vi "Drive Controller.vi"(8 "error in":errorcluster) -> ()   [LabVIEW 2017]
doc: "This VI executes continuously carrying out the current operation and responding to updates or new operation requests. It will often contain the timing or control code that is difficult to place directly in TeleOp. This VI generally opens all sensors and motors and isolates the rest of the robot code from knowing implementation details of how the operations are carried out."
uses:
  <vilib>/Rock Robotics/WPI/Framework/Completion Status.ctl
  Drive Setpoints.ctl
  Drive Operations.ctl
  <vilib>/Rock Robotics/WPI/SafetyOutput/WPI_SafetyOutputConfigMenu.ctl
  <vilib>/Rock Robotics/SystemInterfaces/DIO/FPGA_DIOPWMChannel.ctl
  <vilib>/Rock Robotics/WPI/RobotDrive/WPI_RobotDriveOpen4MotorWithTalonSRX.vi
  Framework/Robot Global Data.vi
  <vilib>/addons/control/pid/pid.llb/PID (DBL).vi
  <vilib>/Rock Robotics/Network Tables/NT Write Numeric Array.vi
  <vilib>/addons/control/pid/NI_PID_pid.lvlib
  <vilib>/Rock Robotics/WPI/ThirdParty/Sensors/ADIS16448 IMU/ADIS16448_IMU.lvlib
panel:
  in  "Interactive Values":T1
  in  "Buttons":cluster{"Execute Cmd":bool, "Abort Cmd":bool}
  out "Command Timing":cluster{"Start Time (ms)":u32, "Iterations":i32}
  out "Status":T3
  out "Setpoints":T4(graph)
  out "Current\nCmd":string
  # "Tip: The graph shows the motor setpoints. It may also be helpful to observe inputs and sensor values.\nYou may also want to display tuning or debugging controls."
  # "Interactive Command: You may fill in the settings for a command\nand schedule it with the Execute button. You can observe and abort\nany command while fine tuning the code for the controller."
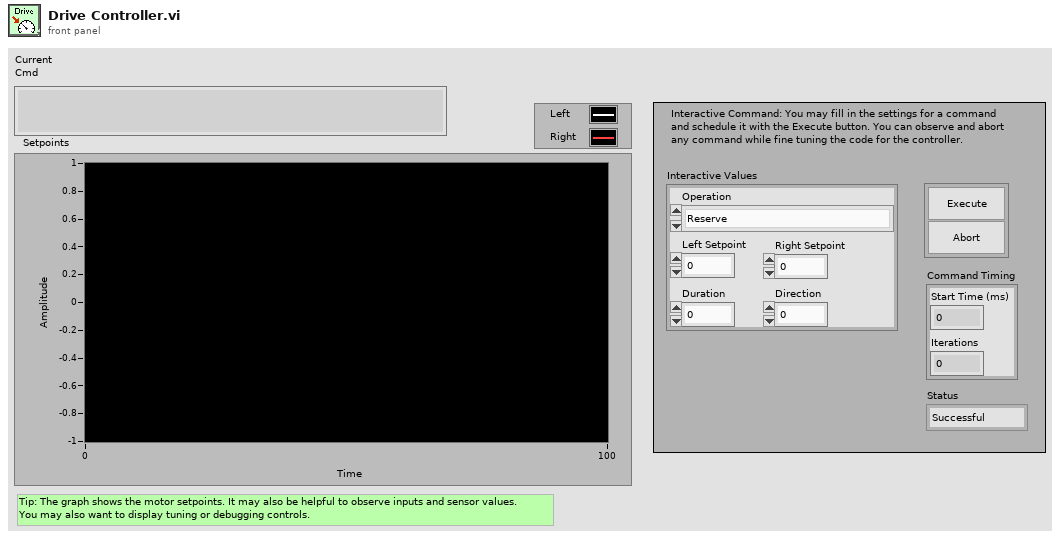
[diagram p1: front panel]
types:
  T1 = typedef "Drive Setpoints.ctl" = cluster{"Operation":T2, "Left Setpoint":dbl, "Right Setpoint":dbl, "Duration":dbl, "Direction":dbl}
  T2 = typedef "Drive Operations.ctl" = enum16{"Reserve", "Read Current", "Immediate", "Drive for Time", "Drive for Distance", "Drive Straight", "Left Turn", "Right Turn", "180 degree Turn", "360 degree Turn"}
  T3 = typedef "Completion Status.ctl" = enum16{"Successful", "Aborted", "Incomplete"}
  T4 = cluster{"Left Setpoint":dbl, "Right Setpoint":dbl}
  T5 = typedef "FPGA_DIOPWMChannel.ctl" = enum8{"PWM 0", "PWM 1", "PWM 2", "PWM 3", "PWM 4", "PWM 5", "PWM 6", "PWM 7", "PWM 8", "PWM 9", "PWM MXP 0", "PWM MXP 1", "PWM MXP 2", "PWM MXP 3", "PWM MXP 4", "PWM MXP 5", "PWM MXP 6", "PWM MXP 7", "PWM MXP 8", "PWM MXP 9", "Invalid"}
  T6 = typedef "WPI_SafetyOutputConfigMenu.ctl" = enum16{"Enable", "Disable"}
  T7 = typedef "WPI_RobotDriveDevRef.ctl" = cluster{"DevStatus":errorcluster, "Motors[]":T8[], "Square Inputs":bool, "Max Output":dbl}
  T8 = typedef "WPI_MotorControlDeviceRef.ctl" = cluster{"DeviceStatus":errorcluster, "Type":T9, "PWM":cluster{"PWM Channel":T5, "DeadBand":T10}, "CAN":cluster{"Device Number":u8, "SetOutput VI Ref":variant, "GetOutput VI Ref":variant, "Enable VI Ref":variant, "Disable VI Ref":variant, "Data":variant}, "Invert":bool, "DIO PWM":cluster{"PWM \"Enable\" Channel":T5, "DIOChannel":T11, "PWM Rate":dbl}}
  T9 = typedef "WPI_MotorControlType.ctl" = enum16{"PWM", "CAN", "DIO PWM"}
  T10 = typedef "WPI_PWMDeadband.ctl" = cluster{"Name":string, "maxPositivePwm":i32, "minPositivePwm":i32, "centerPwm":i32, "maxNegativePwm":i32, "minNegativePwm":i32, "angularRange":u16}
  T11 = typedef "FPGA_DIOChannel.ctl" = enum8{"DIO 0", "DIO 1", "DIO 2", "DIO 3", "DIO 4", "DIO 5", "DIO 6", "DIO 7", "DIO 8", "DIO 9", "DIO MXP 0", "DIO MXP 1", "DIO MXP 2", "DIO MXP 3", "DIO MXP 4", "DIO MXP 5", "DIO MXP 6", "DIO MXP 7", "DIO MXP 8", "DIO MXP 9", "DIO MXP 10", "DIO MXP 11", "DIO MXP 12", "DIO MXP 13", "DIO MXP 14", "DIO MXP 15", "SPI Port CS1", "SPI Port CS2", "SPI Port CS3", "SPI Port MISO", "SPI Port MOSI", "Invalid"}
  T12 = typedef "Command Status Info.ctl" = cluster{"Name":string, "Status":T3, "notifier out":T13}
  T13 = typedef "Completion Notifier.ctl" = refnum<notifier>
  T14 = cluster{"SubSystem Data":T1, cluster{"Start Time (ms)":u32, "Iterations":i32}, cluster{"Command Info":T12, "Description":string, "Default Command":T1, "queue out":refnum<queue>, "Subsystem Name":string}}
  T15 = typedef "ADIS16448_IMU.lvlib/ADI_IMU_ADIS16448_IMUDevRef.ctl" = cluster{"DevStatus":errorcluster, "Handle":i32, "SPI Bus":T16, "Device Found":bool, "Device Ready":bool, "Yaw Axis":enum16{"X", "Y", "Z"}, "AHRS Algorithm":enum16{"Complementary", "Madgwick"}, "Serial":u16, "Lot ID 2":u16, "Lot ID 1":u16, "Bytes Per Sample":u16, "Calibrate On Open?":bool}
  T16 = typedef "spi_bus.ctl" = enum16{"SPI On-Board, CS0", "SPI On-Board, CS1", "SPI On-Board, CS2", "SPI On-Board, CS3", "SPI MXP", "Invalid"}
  T17 = cluster{"proportional gain (Kc)":dbl, "integral time (Ti, min)":dbl, "derivative time (Td, min)":dbl}
  T18 = cluster{"X Angle":dbl, "Y Angle":dbl, "Z Angle":dbl}
  T19 = cluster{"SubSystem Data":T1, cluster{"Start Time (ms)":u32, "Iterations":i32}, "Default Command Arguments":cluster{"Command Info":T12, "Description":string, "Default Command":T1, "queue out":refnum<queue>, "Subsystem Name":string}}
  T20 = cluster{"Don't move motors while reserved":dbl, "Don't move motors while reserved":dbl}
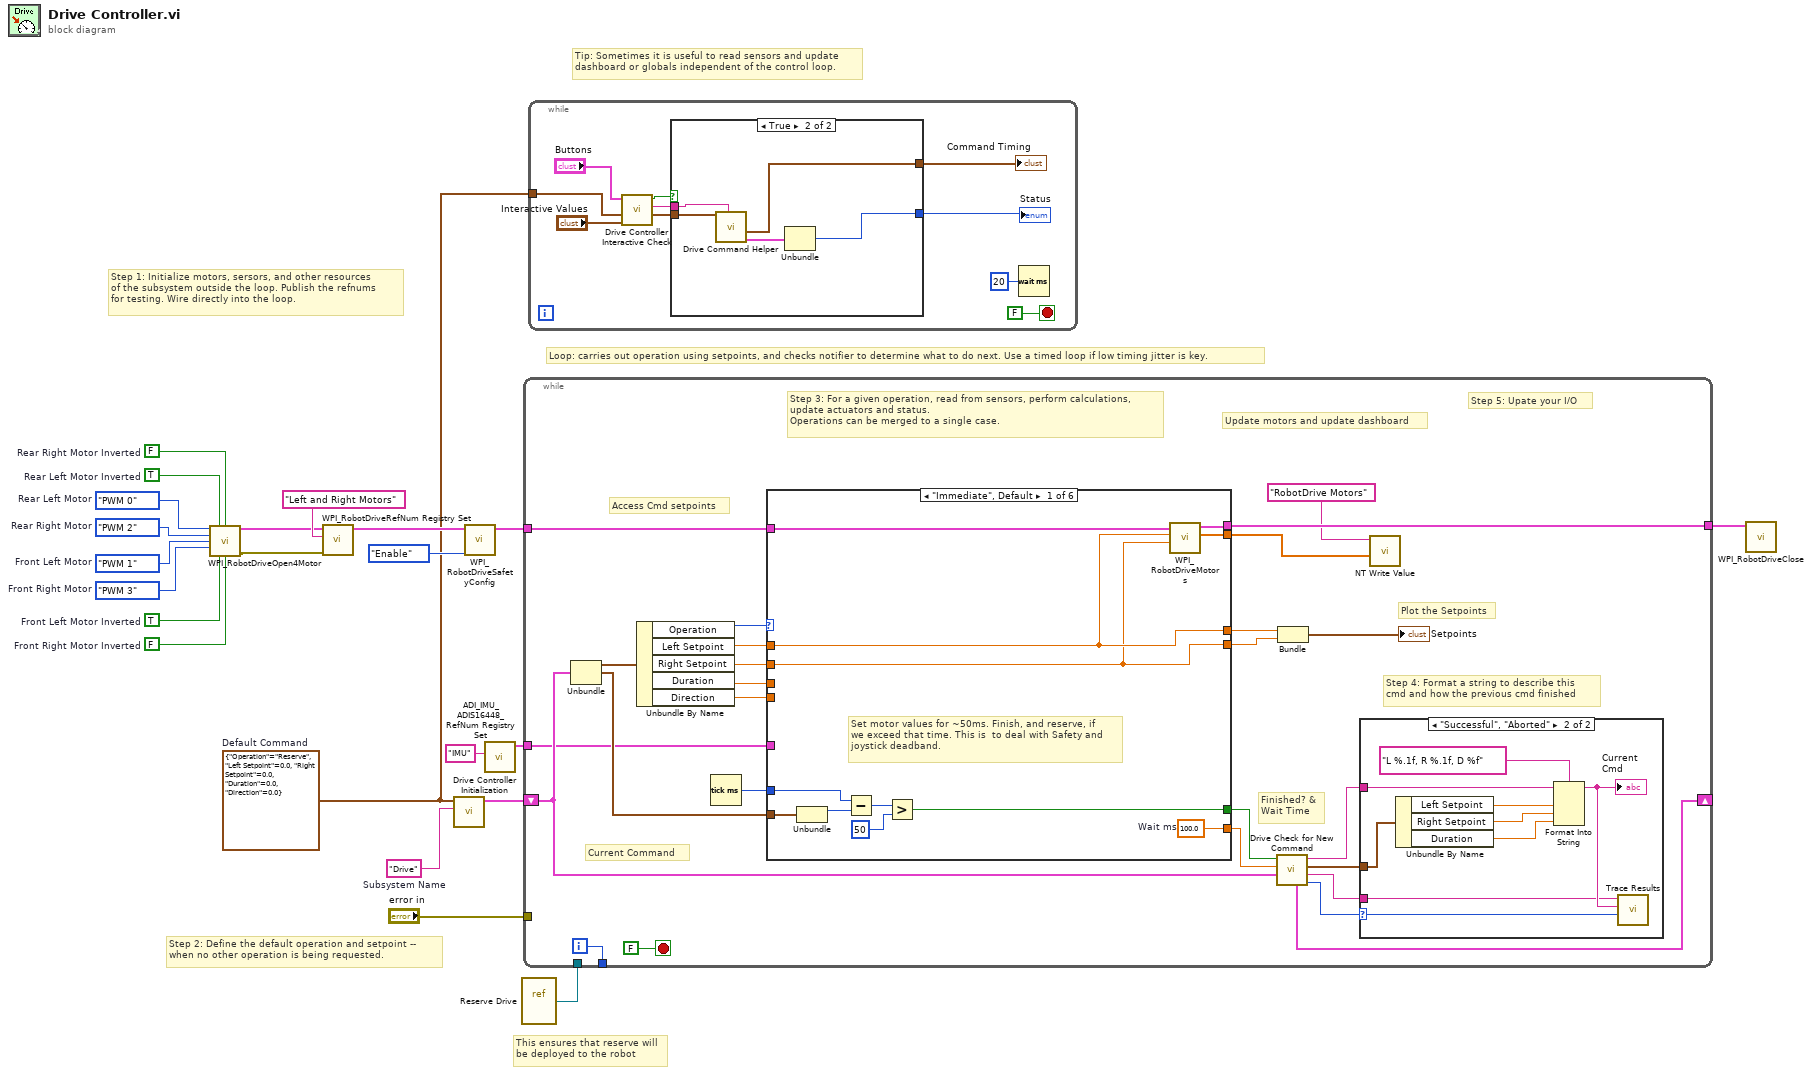
[diagram p0: block diagram]
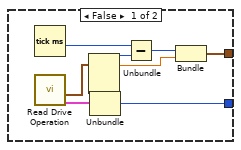
[diagram p2: hidden frame]
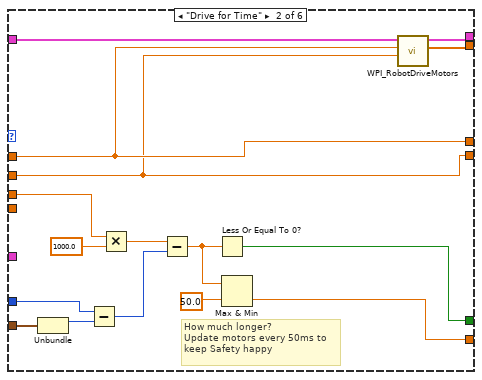
[diagram p4: hidden frame]
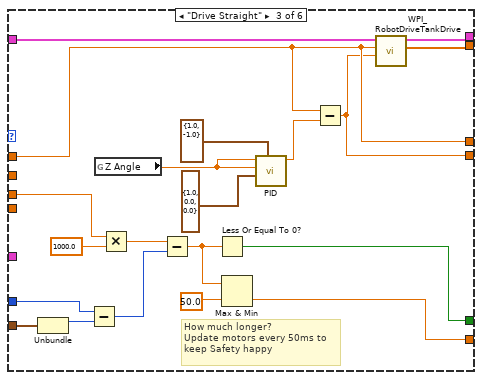
[diagram p5: hidden frame]
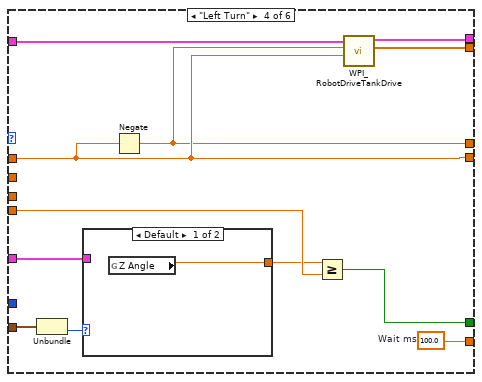
[diagram p6: hidden frame]
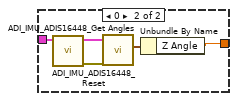
[diagram p7: hidden frame]
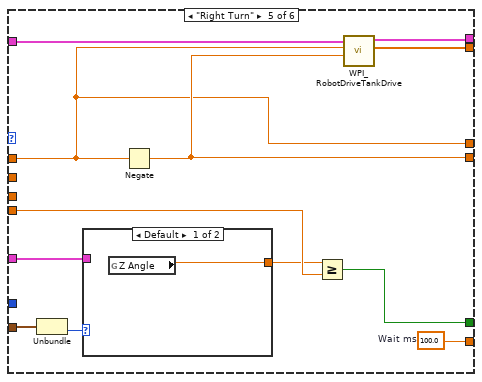
[diagram p8: hidden frame]
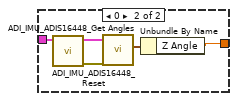
[diagram p9: hidden frame]
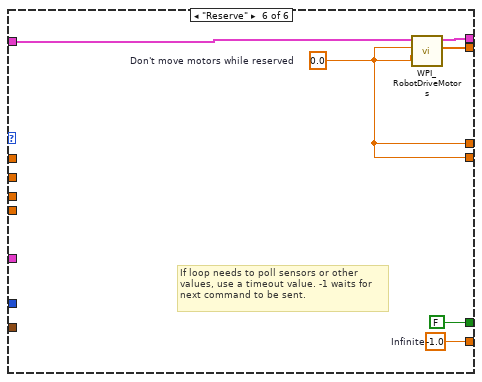
[diagram p10: hidden frame]
diagram:
  w7 = FPGA_DIOPWMChannel."PWM 3"  # Front Right Motor
  w8 = FPGA_DIOPWMChannel."PWM 1"  # Front Left Motor
  w9 = FPGA_DIOPWMChannel."PWM 2"  # Rear Right Motor
  w10 = FPGA_DIOPWMChannel."PWM 0"  # Rear Left Motor
  w11 = FALSE  # Front Right Motor Inverted
  w12 = TRUE  # Front Left Motor Inverted
  w13 = TRUE  # Rear Left Motor Inverted
  w14 = FALSE  # Rear Right Motor Inverted
  w15 = T1 {"Operation"=enum."Reserve", "Left Setpoint"=0.0, "Right Setpoint"=0.0, "Duration"=0.0, "Direction"=0.0}  # Default Command
  w22 = "Drive"  # Subsystem Name
  # "This ensures that reserve will\nbe deployed to the robot"
  # "Tip: Sometimes it is useful to read sensors and update\ndashboard or globals independent of the control loop."
  # "Step 2: Define the default operation and setpoint --\nwhen no other operation is being requested."
  # "Step 1: Initialize motors, sersors, and other resources\nof the subsystem outside the loop. Publish the refnums\nfor testing. Wire directly into the loop."
  # "Loop: carries out operation using setpoints, and checks notifier to determine what to do next. Use a timed loop if low timing jitter is key."
  n1 = call-poly <vilib>:"WPI_RobotDriveOpen4Motor.vi"("Rear Left Motor"=w10, "Rear Left Motor Inverted"=w13, "Rear Right Motor Inverted"=w14, "Rear Right Motor"=w9, "Front Left Motor"=w8, "Front Right Motor"=w7, "Front Left Motor Inverted"=w12, "Front Right Motor Inverted"=w11) -> ("RobotDriveDevRef"=w5:T7, "error out"=w6:errorcluster)  [unwired: 6 in]
  n2 = call <vilib>:"WPI_RobotDriveRefNum Registry Set.vi"("error in (no error)"=w6, "refnum name"="Left and Right Motors", "RobotDriveDevRef"=w5) -> ("RobotDriveDevRef"=w20:T7)  [unwired: 1 in, 7 out]
  n3 = call "Drive Controller Initialization.vi"("Subsystem Name"=w22, "Default Command"=w15) -> ("Current Command"=w17:T14)  [unwired: 9 in]
  n4 = call <vilib>:"WPI_RobotDriveSafetyConfig.vi"("mode"=WPI_SafetyOutputConfigMenu."Enable", "RobotDriveDevRef"=w20) -> ("RobotDriveDevRef"=w4:T7)  [unwired: 8 in, 1 out]
  n5 = call <vilib>:"ADI_IMU_ADIS16448_RefNum Registry Set.vi"("refnum name"="IMU") -> ("ADI IMU DevRef"=w2:T15)  [unwired: 9 in, 1 out]
  n6 = vi-ref "Reserve Drive.vi"() -> (w16:refnum<vi>)
  n7 = while {
    shift-right: [w36] -> _
    shift-left: w17 -> [w29]
    tunnel: [w47] -> _
    tunnel: "error in" -> [_]
    tunnel: w16 -> [_]
    tunnel: w4 -> [w28]
    tunnel: w2 -> [w27]
    tunnel: [w25] -> w1
    i -> [w47]
    stop <- FALSE stop-if-true
    # "Step 5: Upate your I/O"
    # "Step 4: Format a string to describe this\ncmd and how the previous cmd finished"
    # "Current Command"
    # "Update motors and update dashboard"
    # "Plot the Setpoints"
    # "Access Cmd setpoints"
    # "Finished? &\nWait Time"
    # "Step 3: For a given operation, read from sensors, perform calculations,\nupdate actuators and status.\nOperations can be merged to a single case."
    n8 = Unbundle(w29) -> ("SubSystem Data"=w43:T1, w30:cluster{"Start Time (ms)":u32, "Iterations":i32})  [unwired: 1 out]
    n9 = Unbundle By Name(w43) -> ("Operation"=w42:T2, "Left Setpoint"=w41:dbl, "Right Setpoint"=w40:dbl, "Duration"=w39:dbl, "Direction"=w26:dbl)
    n10 = Tick Count (ms)() -> (millisecond timer value=w38:u32)
    n11 = case shown="\"Immediate\", Default" w42 {
      tunnel: [w69 w73 w95 w116 w134 w147] -> w35
      tunnel: [w64 w80 w100 w111 w127 FALSE ("ignore previous (F)")] -> w34
      tunnel: w30 -> [w63 w82 w102 w117 w135 _]
      tunnel: [w61 w79 w91 w106 w131 w144] -> w45
      tunnel: [w60 w78 w89 w107 w132 w144] -> w44
      tunnel: w41 -> [w61 w79 w91 w107 w131 _]
      tunnel: w40 -> [w60 w78 _ _ _ _]
      tunnel: w39 -> [_ w77 w99 _ _ _]
      tunnel: w38 -> [w65 w76 w98 _ _ _]
      tunnel: w28 -> [w62 w72 w88 w115 w133 w145]
      tunnel: w27 -> [_ _ _ w114 w130 _]
      tunnel: w26 -> [_ _ _ w112 w128 _]
      tunnel: [w58 w70 w86 w109 w125 w142] -> w23
      tunnel: [w59 w71 w87 w108 w124 w143] -> w25
      frame "Immediate", Default {
        w69 = 100.0  # Wait ms
        # "Set motor values for ~50ms. Finish, and reserve, if\nwe exceed that time. This is  to deal with Safety and\njoystick deadband."
        n12 = Unbundle(w63) -> ("Start Time (ms)"=w66:u32)  [unwired: 1 out]
        n13 = Subtract(x=w65, y=w66) -> (x-y=w67:u32)
        n14 = Greater?(x=w67, y=u8 50 ("Left Motor")) -> (0:w64:bool)
        n15 = call <vilib>:"WPI_RobotDriveMotors.vi"("RightSpeed"=w60, "LeftSpeed"=w61, "RobotDriveDevRef"=w62) -> ("Motor Values"=w58:dbl[], "RobotDriveDevRef"=w59:T7)  [unwired: 1 in, 6 out]
      }
      frame "Drive for Time" {
        # "How much longer?\nUpdate motors every 50ms to\nkeep Safety happy"
        n16 = Unbundle(w82) -> ("Start Time (ms)"=w81:u32)  [unwired: 1 out]
        n17 = Subtract(x=w76, y=w81) -> (x-y=w85:u32)
        n18 = Multiply(x=w77, y=1000.0) -> (x*y=w84:dbl)
        n19 = Subtract(x=w84, y=w85) -> (x-y=w75:dbl)
        n20 = Less Or Equal To 0?(x=w75) -> (x <= 0?=w80:bool)
        n21 = Max & Min(x=w75, y=50.0) -> (min(x,y)=w73:dbl)  [unwired: 1 out]
        n22 = call <vilib>:"WPI_RobotDriveMotors.vi"("RightSpeed"=w78, "LeftSpeed"=w79, "RobotDriveDevRef"=w72) -> ("Motor Values"=w70:dbl[], "RobotDriveDevRef"=w71:T7)  [unwired: 1 in, 6 out]
      }
      frame "Drive Straight" {
        # "How much longer?\nUpdate motors every 50ms to\nkeep Safety happy"
        n23 = Unbundle(w102) -> ("Start Time (ms)"=w101:u32)  [unwired: 1 out]
        n24 = Subtract(x=w98, y=w101) -> (x-y=w105:u32)
        n25 = global read "Robot Global Data.vi" "Z Angle"() -> (w92:dbl)
        n26 = Multiply(x=w99, y=1000.0) -> (x*y=w104:dbl)
        n27 = Subtract(x=w104, y=w105) -> (x-y=w97:dbl)
        n28 = Less Or Equal To 0?(x=w97) -> (x <= 0?=w100:bool)
        n29 = Max & Min(x=w97, y=50.0) -> (min(x,y)=w95:dbl)  [unwired: 1 out]
        n30 = call-poly <vilib>:"PID.vi"("output range"=cluster{"output high":dbl, "output low":dbl} {"output high"=1.0, "output low"=-1.0}, "PID gains"=T17 {"proportional gain (Kc)"=1.0, "integral time (Ti, min)"=0.0, "derivative time (Td, min)"=0.0}, "process variable"=w92, "setpoint"=w92) -> ("output"=w90:dbl)  [unwired: 6 in, 1 out]
        n31 = Subtract(x=w91, y=w90) -> (x-y=w89:dbl)
        n32 = call <vilib>:"WPI_RobotDriveTankDrive.vi"("Right axis value"=w89, "Left axis value"=w91, "RobotDriveDevRef"=w88) -> ("Motor Values"=w86:dbl[], "RobotDriveDevRef"=w87:T7)  [unwired: 6 in, 1 out]
      }
      frame "Left Turn" {
        w116 = 100.0  # Wait ms
        n33 = Unbundle(w117) -> ("Iterations"=w113:i32)  [unwired: 1 out]
        n34 = case shown="Default" w113 {
          tunnel: w114 -> [_ w121]
          tunnel: [w118 w119] -> w110
          frame Default {
            n35 = global read "Robot Global Data.vi" "Z Angle"() -> (w118:dbl)
          }
          frame 0 {
            n36 = call <vilib>:"ADI_IMU_ADIS16448_Reset.vi"("ADI IMU DevRef"=w121) -> ("error out"=w123:errorcluster, "ADI IMU DevRef Out"=w122:T15)  [unwired: 9 in]
            n37 = call <vilib>:"ADI_IMU_ADIS16448_Get Angles.vi"("error in"=w123, "ADI IMU DevRef"=w122) -> ("IMU Angles Out"=w120:T18)  [unwired: 6 in, 3 out]
            n38 = Unbundle By Name(w120) -> ("Z Angle"=w119:dbl)
          }
        }
        n39 = Negate(x=w107) -> (-x=w106:dbl)
        n40 = Greater Or Equal?(x=w110, y=w112) -> (x >= y?=w111:bool)
        n41 = call <vilib>:"WPI_RobotDriveTankDrive.vi"("Right axis value"=w107, "Left axis value"=w106, "RobotDriveDevRef"=w115) -> ("Motor Values"=w109:dbl[], "RobotDriveDevRef"=w108:T7)  [unwired: 6 in, 1 out]
      }
      frame "Right Turn" {
        w134 = 100.0  # Wait ms
        n42 = Unbundle(w135) -> ("Iterations"=w129:i32)  [unwired: 1 out]
        n43 = case shown="Default" w129 {
          tunnel: w130 -> [_ w139]
          tunnel: [w136 w137] -> w126
          frame Default {
            n44 = global read "Robot Global Data.vi" "Z Angle"() -> (w136:dbl)
          }
          frame 0 {
            n45 = call <vilib>:"ADI_IMU_ADIS16448_Reset.vi"("ADI IMU DevRef"=w139) -> ("error out"=w141:errorcluster, "ADI IMU DevRef Out"=w140:T15)  [unwired: 9 in]
            n46 = call <vilib>:"ADI_IMU_ADIS16448_Get Angles.vi"("error in"=w141, "ADI IMU DevRef"=w140) -> ("IMU Angles Out"=w138:T18)  [unwired: 6 in, 3 out]
            n47 = Unbundle By Name(w138) -> ("Z Angle"=w137:dbl)
          }
        }
        n48 = Negate(x=w131) -> (-x=w132:dbl)
        n49 = Greater Or Equal?(x=w126, y=w128) -> (x >= y?=w127:bool)
        n50 = call <vilib>:"WPI_RobotDriveTankDrive.vi"("Right axis value"=w132, "Left axis value"=w131, "RobotDriveDevRef"=w133) -> ("Motor Values"=w125:dbl[], "RobotDriveDevRef"=w124:T7)  [unwired: 6 in, 1 out]
      }
      frame "Reserve" {
        w144 = 0.0  # Don't move motors while reserved
        w147 = -1.0  # Infinite
        # "If loop needs to poll sensors or other\nvalues, use a timeout value. -1 waits for\nnext command to be sent."
        n51 = call <vilib>:"WPI_RobotDriveMotors.vi"("RightSpeed"=w144, "LeftSpeed"=w144, "RobotDriveDevRef"=w145) -> ("Motor Values"=w142:dbl[], "RobotDriveDevRef"=w143:T7)  [unwired: 1 in, 6 out]
      }
    }
    n52 = call "Drive Check for New Command.vi"("input cluster"=w29, "Wait time (ms)"=w35, "Finished?"=w34) -> ("Completion"=w37:T3, "Subsystem Name"=w31:string, "Current Command"=w32:T1, "Initial Trace String"=w33:string, "Next Command"=w36:T19)  [unwired: 4 in]
    n53 = Bundle("Don't move motors while reserved"=w45, "Don't move motors while reserved"=w44) -> (→"Setpoints":T20)  [unwired: 1 in]
    n54 = case shown="\"Successful\", \"Aborted\"" w37 {
      selector: w37 -> [_ w57]
      tunnel: w33 -> [_ w52]
      tunnel: w32 -> [_ w53]
      tunnel: w31 -> [_ w49]
      frame "Incomplete", Default {
        # "Continuing current command"
      }
      frame "Successful", "Aborted" {
        # "Report and setup for next command"
        n55 = Unbundle By Name(w53) -> ("Left Setpoint"=w55:dbl, "Right Setpoint"=w56:dbl, "Duration"=w50:dbl)
        n56 = Format Into String(format string="L %.1f, R %.1f, D %f", initial string=w52, w55, w56, w50) -> (resulting string=w51:string)  [unwired: 1 in, 1 out]
        "Current\nCmd" <- w51
        n57 = call <vilib>:"Trace Results.vi"("Status of previous command"=w57, "Description"=w51, "Subsystem"=w49) -> ()  [unwired: 9 in]
      }
    }
    n58 = call-poly <vilib>:"NT Write Value.vi"("Numeric Array"=w23, "Name"="RobotDrive Motors") -> ()  [unwired: 9 in, 1 out]
  }
  n59 = while {
    tunnel: w15 -> [w149]
    stop <- FALSE stop-if-true
    n60 = call "Drive Controller Interactive Check.vi"("Interactive Command In"="Interactive Values", "Default Command"=w149, "Buttons"="Buttons") -> ("Interactive Command Out"=w151:T1, "Trace String"=w152:string, "Schedule"=w153:bool)  [unwired: 6 in]
    n61 = case shown="True" w153 {
      tunnel: [w162 w170] -> w154
      tunnel: [w161 w166] -> w155
      tunnel: w152 -> [_ w168]
      tunnel: w151 -> [_ w167]
      frame False {
        n62 = Tick Count (ms)() -> (millisecond timer value=w165:u32)
        n63 = call "Read Drive Operation.vi"() -> ("Command Info"=w159:T12, "SubSystem Data"=w158:T1)  [unwired: 9 in, 1 out]
        n64 = Unbundle(w158) -> ("Operation"=w163:T2, "Left Setpoint"=w160:dbl)  [unwired: 3 out]
        n65 = Unbundle(w159) -> ("Status"=w162:T3)  [unwired: 2 out]
        n66 = Subtract(x=w165, y=w163) -> (x-y=w164:u32)
        n67 = Bundle(w164, "Left Setpoint"=w160) -> (w161:cluster{u32, "Left Setpoint":dbl})  [unwired: 1 in]
      }
      frame True {
        n68 = call "Drive Command Helper.vi"("Description"=w168, "SubSystem Data"=w167) -> ("Command Info Out"=w169:T12, "Command Timing"=w166:cluster{"Start Time (ms)":u32, "Iterations":i32})  [unwired: 7 in, 1 out]
        n69 = Unbundle(w169) -> ("Status"=w170:T3)  [unwired: 2 out]
      }
    }
    "Status" <- w154
    "Command Timing" <- w155
    n70 = Wait (ms)(milliseconds to wait=u32 20) -> ()  [unwired: 1 out]
  }
  n71 = call <vilib>:"WPI_RobotDriveClose.vi"("RobotDriveDevRef"=w1) -> ()  [unwired: 10 in, 1 out]
